vi "Dequeue_Queue.vi"(8 "error in (no error)":errorcluster, 9 "timeout in ms (-1)":i32=-1, 11 "queue In":refnum<queue>) -> (0 "error out":errorcluster, 1 "Data":variant, 2 "Command":string, 3 "queue Out":refnum<queue>)   [LabVIEW 2014, in "Queue_Library.lvlib"]
uses:
  Queue_Library.lvlib
  TypeDef.ctl
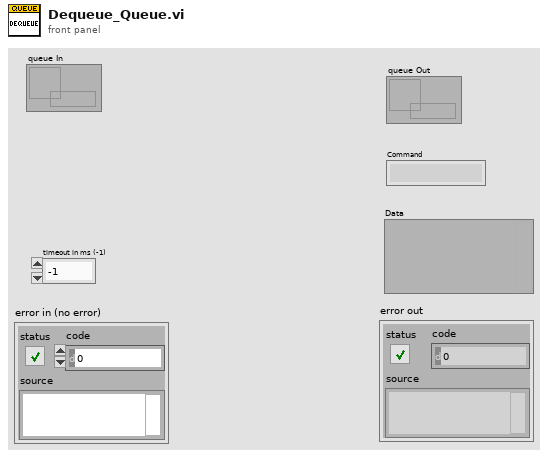
[diagram p1: front panel]
types:
  T1 = typedef "Queue_Library.lvlib/TypeDef.ctl" = cluster{"Command":string, "Data":variant}
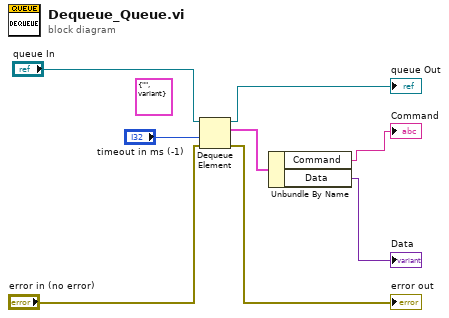
[diagram p0: block diagram]
diagram:
  (unwired) T1 {"Command"="", "Data"=variant} ("Message")
  n1 = Dequeue Element(queue="queue In", timeout in ms (-1)="timeout in ms (-1)", error in (no error)="error in (no error)") -> (queue out=→"queue Out":refnum<queue>, element=w4:T1, error out=→"error out":errorcluster)  [unwired: 1 out]
  n2 = Unbundle By Name(w4) -> ("Command"=→"Command":string, "Data"=→"Data":variant)
